vi "Report.vi"(6 "文件重命名":bool, 7 "文件名称":string, 8 "错误输入（无错误）":errorcluster, 11 "检测结果":bool[][](array[boolean])=[[TRUE]]) -> (0 "error out":errorcluster caption="错误输出", 3 "PRODUCT_VAULE":string)   [LabVIEW 2020]
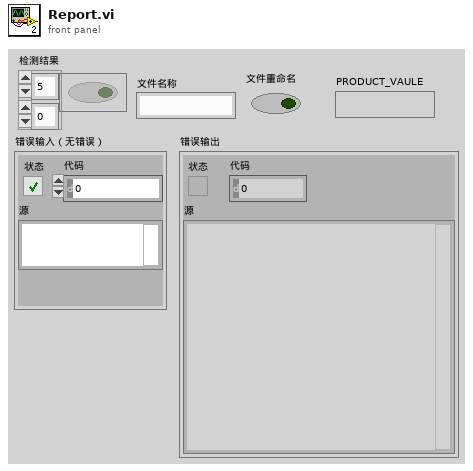
[diagram p1: front panel]
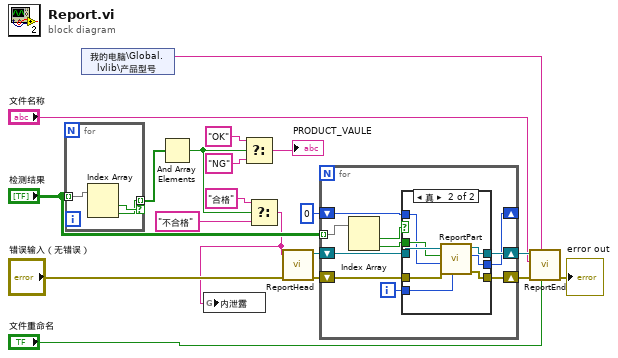
[diagram p0: block diagram]
diagram:
  n1 = for {
    tunnel: [w20] -> w5 mode=indexing if=w21
    tunnel: "检测结果" -> [w22] mode=indexing
    n2 = Index Array(array=w22) -> (element #1=w21:bool, element #2=w20:bool)  [unwired: 2 in]
  }
  n3 = shared-variable "我的电脑\\Global.lvlib\\产品型号"() -> (w2:string)  [unwired: 1 in, 1 out]
  n4 = And Array Elements(Boolean array=w5) -> (logical AND=w6:bool)
  n5 = Select(t="OK", s=w6, f="NG") -> (s? t:f=→"PRODUCT_VAULE":string)
  n6 = Select(t="合格", s=w6, f="不合格") -> (s? t:f=w1:string)
  n7 = global write "检测结果.vi" "内泄露"(w1) -> ()
  n8 = call "ReportHead.vi"("error in (no error)"="错误输入（无错误）", "产品状态"=w1) -> ("error out"=w18:errorcluster, "report out"=w19:refnum<class "NI_report.lvclass">)  [unwired: 8 in]
  n9 = for {
    shift-right: [w30] -> w17
    shift-left: w19 -> [w32]
    shift-right: [w29] -> w16
    shift-left: w18 -> [w31]
    tunnel: "检测结果" -> [w25] mode=indexing
    shift-right: [w26] -> _
    shift-left: 0 ("索引OUT") -> [w27]
    i -> [w28]
    n10 = Index Array(array=w25) -> (element #1=w24:bool, element #2=w23:bool)  [unwired: 2 in]
    n11 = case shown="真" w24 {
      tunnel: w32 -> [w34 w41]
      tunnel: w31 -> [w35 w42]
      tunnel: [w34 w40] -> w30
      tunnel: [w35 w38] -> w29
      tunnel: w28 -> [_ w43]
      tunnel: w23 -> [_ w37]
      tunnel: w27 -> [w33 w36]
      tunnel: [w33 w39] -> w26
      frame False {
      }
      frame True {
        n12 = call "ReportPart.vi"("试验项目"=w43, "error in"=w42, "索引IN"=w36, "合格"=w37, "report in"=w41) -> ("error out 2"=w38:errorcluster, "索引OUT"=w39:i32, "report out"=w40:refnum<class "NI_report.lvclass">)  [unwired: 4 in]
      }
    }
  }
  n13 = call "ReportEnd.vi"("文件重命名"="文件重命名", "产品型号"=w2, "error in (no error)"=w16, "文件名称"="文件名称", "report in"=w17) -> ("error out"=→"error out":errorcluster)  [unwired: 6 in]
